vi "GetCurrentPVRequest.vi"() -> (3 "Request":u8[](array[numeric]))   [LabVIEW 2017]
uses:
  <instrlib>/Samwontech TEMP2xxx/Samwontech TEMP2xxx.lvlib
panel:
  out "Request":string
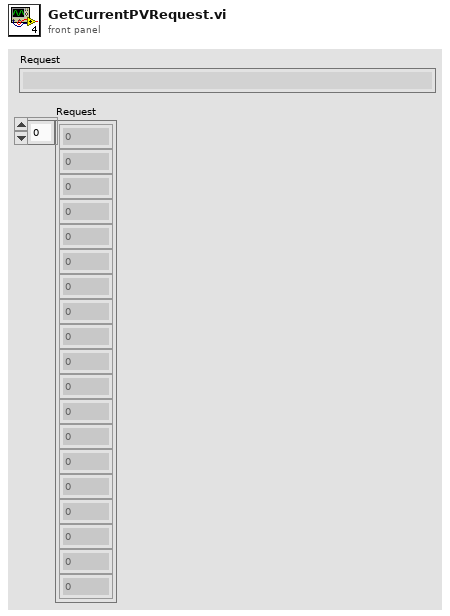
[diagram p1: front panel]
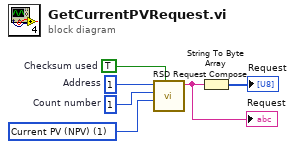
[diagram p0: block diagram]
diagram:
  w3 = u32 1 items=["Current PV (NPV)"=1, "Operation Control (COM.OPMODE)"=102, "Set Point on FIX operation (FIX.TSP)"=104, "Operation Mode (OP.MODE)"=106] ("D-Registers Map")
  w5 = u8 1  # Count number
  w4 = u8 1  # Address
  w6 = TRUE  # Checksum used
  n1 = call <instrlib>:"RSD Request Compose.vi"("Checksum used"=w6, "D-register number"=w3, "Count number"=w5, "Address"=w4) -> ("Request"=w2:string)  [unwired: 6 in, 1 out]
  "Request" <- w2
  n2 = String To Byte Array(string=w2) -> (unsigned byte array=→"Request":u8[])
